vi "Append Control Image to Report.vi"(0 "report in":refnum<class "NI_Excel.lvclass">, 1 "alignment (default)":T2, 2 "image file type (.jpg)":enum16{".jpg", ".png"}(ring), 5 "image depth":T1=3 items=["B&W", "4 bits", "8 bits", "24 bits"], 7 "ctrl reference":refnum<vi>, 9 "description":string, 11 "error in (no error)":errorcluster, 12 "MS Office parameters":T3) -> (4 "report out":refnum<class "NI_Excel.lvclass">, 8 "start out (Word)":i32, 10 "end out (Word)":i32, 15 "error out":errorcluster)   [LabVIEW 2020, in "NI_Excel.lvclass"]
doc: "Creates an image of the front panel object specified in <B>Ctrl Reference</B> and appends it to a report."
uses:
  <vilib>/Utility/NIReport.llb/Excel/NI_Excel.lvclass
  <vilib>/Utility/NIReport.llb/HTML Report Image Alignment.ctl
  <vilib>/Utility/NIReport.llb/image depth.ctl
  <vilib>/Utility/NIReport.llb/Excel/NI_Excel.lvclass/NI_Excel.ctl
  <vilib>/addons/_office/NI_ReportGenerationToolkit.lvlib
  <vilib>/Utility/NIReport.llb/NI_ReportGenerationCore.lvlib
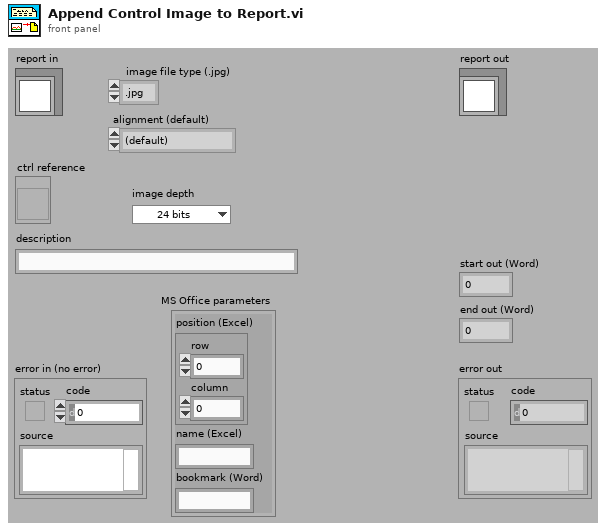
[diagram p1: front panel]
types:
  T1 = typedef "NI_ReportGenerationCore.lvlib/image depth.ctl" = u16
  T2 = typedef "NI_ReportGenerationCore.lvlib/HTML Report Image Alignment.ctl" = enum16{"(default)", "LEFT", "RIGHT", "TOP", "TEXTTOP", "MIDDLE", "ABSMIDDLE", "BASELINE", "BOTTOM", "ABSBOTTOM"}
  T3 = cluster{"position (Excel)":cluster{"row":i32, "column":i32}, "name (Excel)":string, "bookmark (Word)":string}
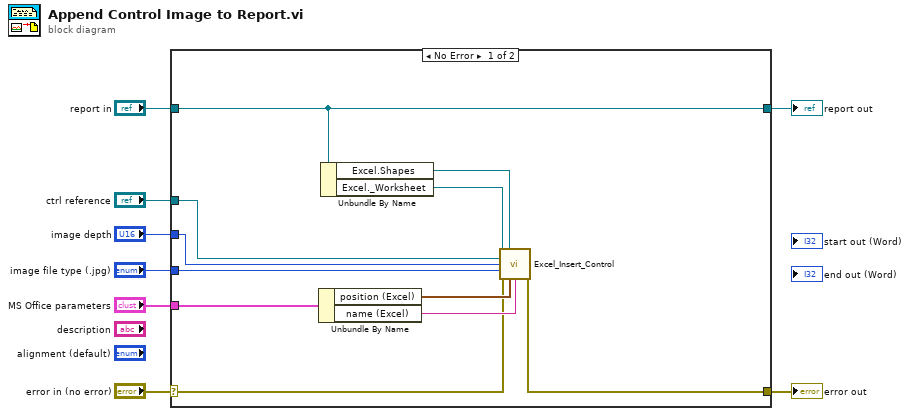
[diagram p0: block diagram]
diagram:
  n1 = case shown="No Error" "error in (no error)" {
    selector: "error in (no error)" -> [w14 w21]
    tunnel: [w13 w21] -> w7
    tunnel: [w15 w20] -> w5
    tunnel: "report in" -> [w15 w20]
    tunnel: "MS Office parameters" -> [w12 _]
    tunnel: "image file type (.jpg)" -> [w11 _]
    tunnel: "ctrl reference" -> [w10 _]
    tunnel: "image depth" -> [w9 _]
    frame No Error {
      n2 = Unbundle By Name(w12) -> ("position (Excel)"=w18:cluster{"row":i32, "column":i32}, "name (Excel)"=w19:string)
      n3 = Unbundle By Name(w15) -> ("Excel.Shapes"=w16:refnum<k7>, "Excel._Worksheet"=w17:refnum<k7>)
      n4 = call <vilib>:"Excel_Insert_Control.vi"("Worksheet"=w17, "Excel.Shapes"=w16, "Ctl Refnum"=w10, "image depth"=w9, "image file type(.jpg)"=w11, "error in (no error)"=w14, "Position (Excel)"=w18, "name"=w19) -> ("error out"=w13:errorcluster)  [unwired: 7 out]
    }
    frame Error {
    }
  }
  "error out" <- w7
  "report out" <- w5
